vi "test2_2xq - renew.vi"() -> ()   [LabVIEW 2018]
uses:
  <vilib>/imath/engines/lvmath/Plug In/_Char/NIMS_CH_character datatype.ctl
  <vilib>/imath/engines/lvmath2/RunTimeEngine/RangeToken/NIMS_Range.vi
  <instcachedir>/0/NIMS_Range_846134F467D14A349F7C6CCEF459CDB2.lvgen/NIMS_Range_846134F467D14A349F7C6CCEF459CDB2_000.vi
  <vilib>/imathl/engines/lvmath/Functions/Error Handling/Create Error.vi
  <vilib>/imath/engines/lvmath/Plug In/_Char/NIMS_CH_Character RV to String.vi
  <vilib>/imath/engines/lvmath2/RunTimeEngine/BuiltInFunctions/random/NIMS_random.vi
  <vilib>/imath/engines/lvmath2/RunTimeEngine/BuiltInFunctions/length/NIMS_length(GV).vi
  <instcachedir>/0/NIMS_length(GV)_08A3D13377FD4E4B96F5795FBF3698FA.lvgen/NIMS_length(GV)_08A3D13377FD4E4B96F5795FBF3698FA_000.vi
  <vilib>/imath/engines/lvmath2/RunTimeEngine/IndexRead/NIMS M(S).vi
  <instcachedir>/0/NIMS M(S)_B826C018497E4940AE96BD27B540B6FB.lvgen/NIMS M(S)_B826C018497E4940AE96BD27B540B6FB_000.vi
  <vilib>/imath/engines/lvmath2/RunTimeEngine/ArithmeticOperatorToken/NIMS_ArithmeticOperator_plus.vi
  <instcachedir>/0/NIMS_ArithmeticOperator_plus_DE670E32103C4C10ADF2A97367172B30.lvgen/NIMS_ArithmeticOperator_plus_DE670E32103C4C10ADF2A97367172B30_004.vi
  <vilib>/imath/engines/lvmath2/RunTimeEngine/ErrorHandling/NIMS_Create Error From Enums.vi
  <vilib>/imath/engines/lvmath2/RunTimeEngine/BuiltInFunctions/randnormal/NIMS_randnormal(1,I32).vi
  <vilib>/imath/engines/lvmath2/RunTimeEngine/ErrorHandling/NIMS_Error From Error Code.vi
  <vilib>/imath/engines/lvmath/Functions/Error Handling/MergeErrorsWrapper.vi
  <vilib>/imath/engines/lvmath2/RunTimeEngine/BuiltInFunctions/reshapemx/NIMS_[GM]_reshapemx.vi
  <instcachedir>/0/NIMS_[GM]_reshapemx_BAE328BFC7D2442A9AA111F51FBA2CAD.lvgen/NIMS_[GM]_reshapemx_BAE328BFC7D2442A9AA111F51FBA2CAD_000.vi
  <vilib>/imath/engines/lvmath2/RunTimeEngine/ArithmeticOperatorToken/NIMS_ArithmeticOperator_multmx(RV,M).vi
  <instcachedir>/0/NIMS_ArithmeticOperator_multmx(RV,M)_D6CB063A8E334F19B90764CB3E9B6C99.lvgen/NIMS_ArithmeticOperator_multmx(RV,M)_D6CB063A8E334F19B90764CB3E9B6C99_002.vi
  <vilib>/imath/engines/lvmath2/RunTimeEngine/IndexRead/NIMS V(R3).vi
  <instcachedir>/0/NIMS V(R3)_BB7B7B2F47B844E7B6C44853B6A6C035.lvgen/NIMS V(R3)_BB7B7B2F47B844E7B6C44853B6A6C035_000.vi
  <vilib>/imath/engines/lvmath2/RunTimeEngine/BuiltInFunctions/crosscorr/NIMS_crosscorr(GM,Str).vi
  <instcachedir>/0/NIMS_crosscorr(GM,Str)_B40E69E1A515490ABE9B33FB59F56A52.lvgen/NIMS_crosscorr(GM,Str)_B40E69E1A515490ABE9B33FB59F56A52_000.vi
  <vilib>/imath/engines/lvmath2/RunTimeEngine/BuiltInFunctions/fft/NIMS_fft(GM).vi
  <instcachedir>/0/NIMS_fft(GM)_4D6538E03936427980510B9710B4978C.lvgen/NIMS_fft(GM)_4D6538E03936427980510B9710B4978C_000.vi
  <vilib>/imath/engines/lvmath2/RunTimeEngine/BuiltInFunctions/abs/NIMS_abs(signed).vi
  <instcachedir>/0/NIMS_abs(signed)_C4FCB8E6058B49B797C7C8D53CA5F6EC.lvgen/NIMS_abs(signed)_C4FCB8E6058B49B797C7C8D53CA5F6EC_003.vi
  <vilib>/imath/engines/lvmath2/RunTimeEngine/BuiltInFunctions/length/NIMS_length(GM).vi
  <instcachedir>/0/NIMS_length(GM)_47CEC356FCE0482D9BA47DC61C99F2C7.lvgen/NIMS_length(GM)_47CEC356FCE0482D9BA47DC61C99F2C7_005.vi
  <vilib>/imath/engines/lvmath2/RunTimeSupport/NIMS_Error if Not Equal.vi
  <instcachedir>/0/NIMS_Error if Not Equal_C77461FADD9B4AE6B0EA3ED6E3A6D94D.lvgen/NIMS_Error if Not Equal_C77461FADD9B4AE6B0EA3ED6E3A6D94D_001.vi
  <vilib>/imath/engines/lvmath2/RunTimeEngine/IndexRead/NIMS M(V).vi
  <instcachedir>/0/NIMS M(V)_948FAC22C1C943948B75DA6190348614.lvgen/NIMS M(V)_948FAC22C1C943948B75DA6190348614_004.vi
  <vilib>/imath/engines/lvmath2/RunTimeEngine/BuiltInFunctions/max/1 input/NIMS_max(CM).vi
  <instcachedir>/0/NIMS_max(CM)_7C352D5305924AD7A6AA4FE491F9CF6D.lvgen/NIMS_max(CM)_7C352D5305924AD7A6AA4FE491F9CF6D_000.vi
  <vilib>/imath/engines/lvmath2/RunTimeEngine/IndexRead/NIMS M(S,S).vi
  <instcachedir>/0/NIMS M(S,S)_AC51E74150A542F7991B9634C66F3096.lvgen/NIMS M(S,S)_AC51E74150A542F7991B9634C66F3096_002.vi
  <vilib>/imath/engines/lvmath2/RunTimeEngine/IndexReplace/NIMS M(R2)=M.vi
  <instcachedir>/0/NIMS M(R2)=M_FCAA25EC0B4B43F883DFBC78DC36B741.lvgen/NIMS M(R2)=M_FCAA25EC0B4B43F883DFBC78DC36B741_000.vi
  <vilib>/imath/engines/lvmath2/RunTimeEngine/NodeEndStatement/NIMS_NodeEndStatement_Get Vector.vi
  <instcachedir>/0/NIMS_NodeEndStatement_Get Vector_329D0992E87F49F089135171B7FC9327.lvgen/NIMS_NodeEndStatement_Get Vector_329D0992E87F49F089135171B7FC9327_003.vi
  <vilib>/imath/engines/lvmath2/RunTimeEngine/NodeEndStatement/NIMS_NodeEndStatement_Output.vi
  <instcachedir>/0/NIMS_NodeEndStatement_Output_53EC0D466D134D7ABD903AC30B43404B.lvgen/NIMS_NodeEndStatement_Output_53EC0D466D134D7ABD903AC30B43404B_011.vi
  <instcachedir>/0/NIMS_NodeEndStatement_Output_53EC0D466D134D7ABD903AC30B43404B.lvgen/NIMS_NodeEndStatement_Output_53EC0D466D134D7ABD903AC30B43404B_005.vi
  <vilib>/imath/engines/lvmath2/RunTimeEngine/ErrorHandling/NIMS_Finalize Error.vi
panel:
  out "Waveform Graph":dbl[](graph)
  out "In2":dbl
  out "In1":dbl
  out "Sx1":cluster{"BIN":dbl[], "N":dbl[]}(graph)
  in  "fs":dbl=1000.0
  in  "N":dbl=1024.0
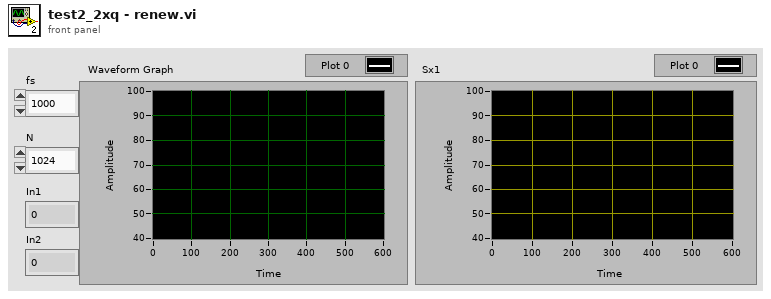
[diagram p1: front panel]
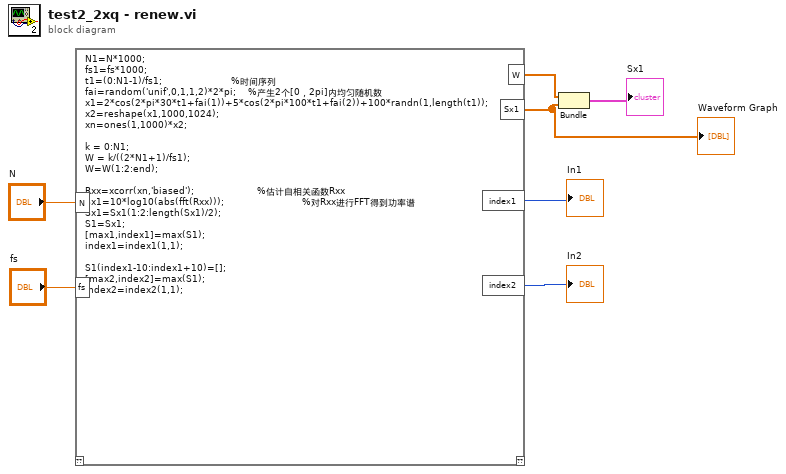
[diagram p0: block diagram]
diagram:
  n1 = mathscript code="N1=N*1000;\nfs1=fs*1000;\nt1=(0:N1-1)/fs1;                       %时间序列\nfai=random('unif',0,1,1,2)*2*pi;    %产生2个[0，2pi]内均匀随机数\nx1=2*cos(2*pi*30*t1+fai(1))+5*cos(2*pi*100*t1+fai(2))+100*randn(1,length(t1));\nx2=reshape(x1,1000,1024);\nxn=ones(1,1000)*x2; \n\nk = 0:N1;\nW = k/((2*N1+1)/fs1);\nW=W(1:2:end);\n\nRxx=xcorr(xn,'biased');                     %估计自相关函数Rxx\nSx1=10*log10(abs(fft(Rxx)));                          %对Rxx进行FFT得到功率谱\nSx1=Sx1(1:2:length(Sx1)/2);\nS1=Sx1;\n[max1,index1]=max(S1);\nindex1=index1(1,1);\n\nS1(index1-10:index1+10)=[];\n[max2,index2]=max(S1);\nindex2=index2(1,1);"("N"="N", "fs"="fs") -> ("Sx1"=w1:dbl[], "W"=w4:dbl[], "index1"=→"In1":i32, "index2"=→"In2":i32)  [unwired: 1 in, 1 out]
  "Waveform Graph" <- w1
  n2 = Bundle("W"=w4, "Sx1"=w1) -> (→"Sx1":cluster{"W":dbl[], "Sx1":dbl[]})  [unwired: 1 in]
